vi "FA_SetAgentConfig.vi"(8 "Error In":errorcluster, 11 "AgentConfig":T1) -> (0 "Error Out":errorcluster)   [LabVIEW 2013, in "FA_AgentConfig.lvlib"]
uses:
  FA_AgentConfig.lvlib
  FA_AgentConfig.ctl
  FA_LocalStore API/source/VI Source/FA_LSSpecialTypes.ctl
  FA_LocalStore API/source/VI Source/FA_LocalStore.lvlib
  FA_NativeTypes API/source/VI Source/FA_NativeTypes.lvlib
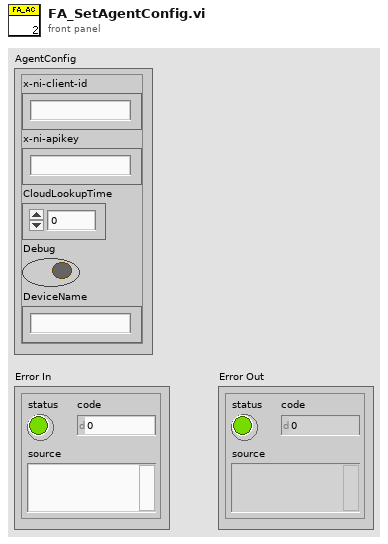
[diagram p1: front panel]
types:
  T1 = typedef "FA_AgentConfig.lvlib/FA_AgentConfig.ctl" = cluster{"x-ni-client-id":string, "x-ni-apikey":string, "CloudLookupTime":u32, "Debug":bool, "DeviceName":string}
  T2 = typedef "FA_LocalStore.lvlib/FA_LSSpecialTypes.ctl" = string
  T3 = typedef "FA_NativeTypes.lvlib/FA_Config.ctl" = cluster{"Id":string, "Name":T2, "Parameter":cluster{"Name":string, "Value":string}[], "Account":string, "CreateDate":string, "LastModified":string}
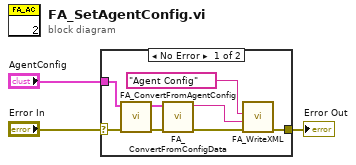
[diagram p0: block diagram]
diagram:
  n1 = case shown="No Error" "Error In" {
    selector: "Error In" -> [w5 w12]
    tunnel: [w6 w12] -> w2
    tunnel: "AgentConfig" -> [w4 _]
    frame No Error {
      n2 = call "FA_ConvertFromAgentConfig.vi"("Error In"=w5, "AgentConfig"=w4) -> ("Error Out"=w10:errorcluster, "Config"=w11:T3)  [unwired: 8 in]
      n3 = call "FA_ConvertFromConfigData.vi"("Error In"=w10, "Config"=w11) -> ("Error Out"=w9:errorcluster, "XML String"=w7:string)  [unwired: 8 in]
      n4 = call "FA_WriteXML.vi"("Error In"=w9, "XML String"=w7, "Special Type"=T2 "Agent Config") -> ("Error Out"=w6:errorcluster)  [unwired: 6 in]
    }
    frame Error {
    }
  }
  "Error Out" <- w2
